vi "polling the value of boolean control.vi"() -> ()   [LabVIEW 2016]
panel:
  in  "Do some work":bool
  out "Iteration number":i32
  out "Work done":i32
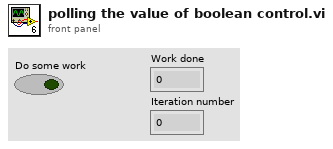
[diagram p1: front panel]
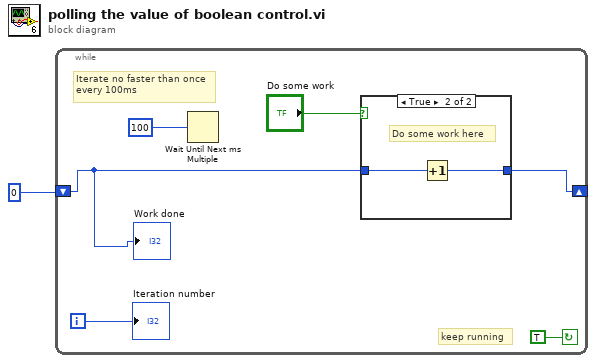
[diagram p0: block diagram]
diagram:
  n1 = while {
    shift-right: [w6] -> _
    shift-left: 0 -> [w5]
    i -> [w4]
    stop <- TRUE continue-if-true
    # "Iterate no faster than once\nevery 100ms"
    # "keep running"
    n2 = Wait Until Next ms Multiple(millisecond multiple=100) -> ()  [unwired: 1 out]
    n3 = case shown="True" "Do some work" {
      tunnel: w5 -> [w8 w10]
      tunnel: [w8 w9] -> w6
      frame False {
      }
      frame True {
        # "Do some work here"
        n4 = Increment(x=w10) -> (x+1=w9:i32)
      }
    }
    "Work done" <- w5
    "Iteration number" <- w4
  }
